vi "call_MB_TCP.vi"(5 "Status Reference":T3, 6 "N":i32, 7 "Data Reference":T2, 8 "error in":errorcluster, 9 "timeouts":T1, 10 "Module Name":string="MB_TCP_ZERO.vi") -> (0 "error out":errorcluster, 3 "reference":refnum<vi>)   [LabVIEW 2019]
panel:
  # "VI Name:\nPurpose: Dynamically calls *.vi"
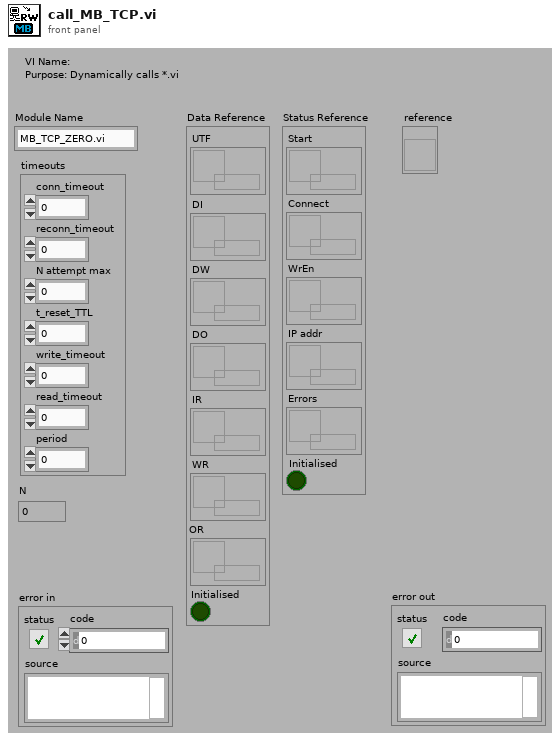
[diagram p1: front panel]
types:
  T1 = cluster{"conn_timeout":i32, "reconn_timeout":u32, "N attempt max":i32, "t_reset_TTL":u32, "write_timeout":i32, "read_timeout":i32, "period":u32}
  T2 = cluster{"UTF":refnum<data-value>, "DI":refnum<data-value>, "DW":refnum<data-value>, "DO":refnum<data-value>, "IR":refnum<data-value>, "WR":refnum<data-value>, "OR":refnum<data-value>, "Initialised":bool}
  T3 = cluster{"Start":refnum<data-value>, "Connect":refnum<data-value>, "WrEn":refnum<data-value>, "IP addr":refnum<data-value>, "Errors":refnum<data-value>, "Initialised":bool}
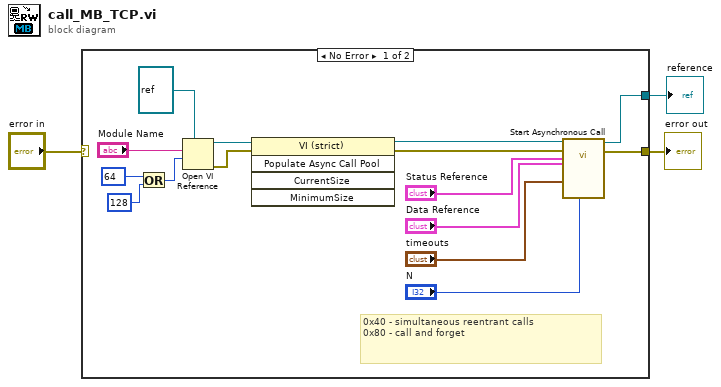
[diagram p0: block diagram]
diagram:
  n1 = case shown="No Error" "error in" {
    selector: "error in" -> [_ w19]
    tunnel: [w9 w19] -> w3
    tunnel: [w10 _] -> w1
    frame No Error {
      # "0x40 - simultaneous reentrant calls\n0x80 - call and forget"
      n2 = Or(x=64 ("options"), y=128 ("options")) -> (x .or. y?=w16:i32)
      n3 = Open VI Reference(type specifier VI Refnum (for type only)=refnum<vi> refnum, vi path="Module Name", options=w16) -> (vi reference=w8:refnum<vi>, error out=w7:errorcluster)  [unwired: 3 in]
      n4 = invoke class="VI (strict)" method="Populate Async Call Pool"(reference=w8, error in=w7) -> (reference out=w6:refnum<vi>, error out=w5:errorcluster)  [unwired: 3 in, 3 out]
      n5 = call-by-ref "Start Asynchronous Call"(reference=w6, error in=w5, "Status Reference"="Status Reference", "N"="N", "Data Reference"="Data Reference", "timeouts"="timeouts") -> (reference out=w10:refnum<vi>, error out=w9:errorcluster)  [unwired: 5 in, 3 out]
    }
    frame Error {
    }
  }
  "error out" <- w3
  "reference" <- w1
